vi "step7 TestIfAllCornersSolved.vi"(11 "cube in":T1) -> (2 "all corners solved?":bool, 3 "cube out":T1)   [LabVIEW 2011]
uses:
  Typedef/cube.ctl
  Typedef/face.ctl
  Typedef/cube rotate direction.ctl
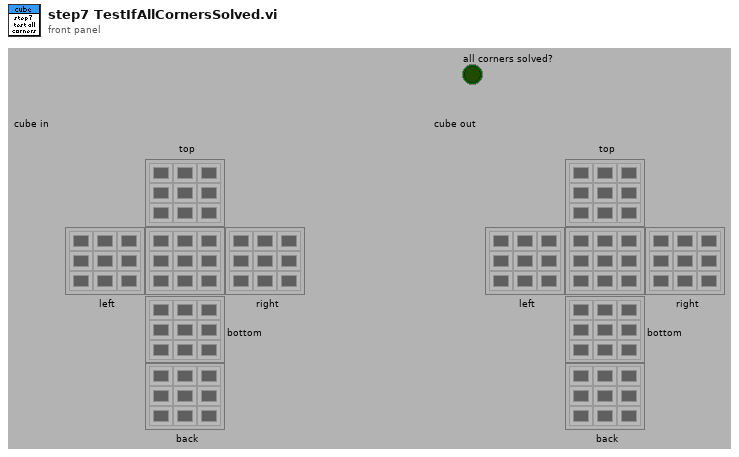
[diagram p1: front panel]
types:
  T1 = typedef "cube.ctl" = cluster{"top":T2, "left":T2, "right":T2, "bottom":T2, "back":T2, "front":T2}
  T2 = typedef "face.ctl" = u32[][]
  T3 = typedef "cube rotate direction.ctl" = enum16{"up", "down", "left", "right"}
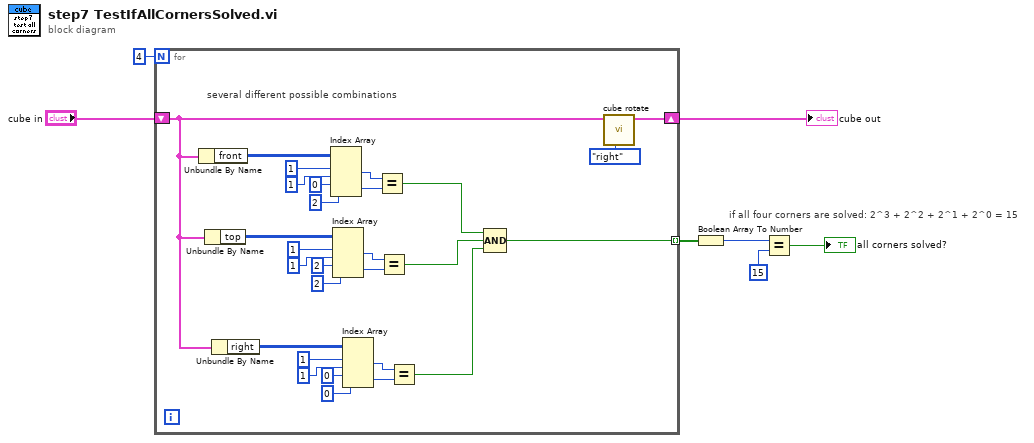
[diagram p0: block diagram]
diagram:
  # "if all four corners are solved: 2^3 + 2^2 + 2^1 + 2^0 = 15"
  n1 = for {
    N: 4 -> [_]
    shift-right: [w33] -> w7
    shift-left: "cube in" -> [w12]
    tunnel: [w8] -> w1 mode=indexing
    # "several different possible combinations"
    n2 = Unbundle By Name(w12) -> ("front"=w32:T2)
    n3 = Unbundle By Name(w12) -> ("top"=w22:T2)
    n4 = Unbundle By Name(w12) -> ("right"=w17:T2)
    n5 = Index Array(array=w32, index (row) #1=1 ("index (row)"), index (col) #1=1 ("disabled index (col)"), index (row) #2=0 ("index (row)"), index (col) #2=2 ("disabled index (col)")) -> (element #1=w28:u32, element #2=w29:u32)
    n6 = Index Array(array=w22, index (row) #1=1 ("index (row)"), index (col) #1=1 ("disabled index (col)"), index (row) #2=2 ("index (row)"), index (col) #2=2 ("disabled index (col)")) -> (element #1=w26:u32, element #2=w25:u32)
    n7 = Index Array(array=w17, index (row) #1=1 ("index (row)"), index (col) #1=1 ("disabled index (col)"), index (row) #2=0 ("index (row)"), index (col) #2=0 ("disabled index (col)")) -> (element #1=w13:u32, element #2=w14:u32)
    n8 = Equal?(x=w28, y=w29) -> (x = y?=w11:bool)
    n9 = Equal?(x=w26, y=w25) -> (x = y?=w10:bool)
    n10 = Equal?(x=w13, y=w14) -> (x = y?=w9:bool)
    n11 = Compound Arithmetic op=AND(w11, w10, w9) -> (w8:bool)
    n12 = call "cube rotate.vi"("cube rotation direction"=cube_rotate_direction."right", "cube in"=w12) -> ("cube out"=w33:T1)  [unwired: 8 in, 1 out]
  }
  "cube out" <- w7
  n13 = Boolean Array To Number(Boolean array=w1) -> (number=w4:u32)
  n14 = Equal?(x=w4, y=u32 15) -> (x = y?=→"all corners solved?":bool)
